vi "Periodic Tasks.vi"(8 "error in":errorcluster) -> ()   [LabVIEW 2017]
doc: "This VI runs in parallel to other tasks. It can contain as many user-defined periodic loops as you need. These can carry out PID or other sorts of timed response."
uses:
  <vilib>/Rock Robotics/WPI/Utilities/WPI_GetSetVariantRefNum.vi
  Robot Global Data.vi
  <vilib>/addons/control/pid/pid.llb/PID (DBL).vi
  <vilib>/Rock Robotics/WPI/RobotDrive/WPI_RobotDriveMecanumDrive_Cartesian.vi
  globals.vi
  <vilib>/addons/control/pid/NI_PID_pid.lvlib
  <vilib>/Rock Robotics/WPI/ThirdParty/Sensors/navX/_TypeDefs/FRIC_navX_DeviceNumbersTypeDef.ctl
panel:
  out "Shoulder Low Home":bool
  out "Wrist Low Home":bool
  out "Wrist High Home":bool
  out "X and Y  axis":cluster{"Distance":dbl, "Distance":dbl}(graph)={"Distance"=0.0, "Distance"=-36.75}
  out "Proxy":dbl(graph)=0.412597614
  in  "PID gains":T1={"proportional gain (Kc)"=0.015, "integral time (Ti, min)"=0.00357142, "derivative time (Td, min)"=0.00089286} {"derivative time (Td, min)" step=1e-05 format="%.9f"; "integral time (Ti, min)" step=1e-05 format="%.9f"; "proportional gain (Kc)" step=0.05 format="%.9f"}
  in  "Wrist Encoder Recording Data":cluster{dbl, u32}[](array[cluster])=[{0.0, 106}, {0.0, 200}, {0.0, 304}, {0.0, 400}, {16.75, 500}, {68.5, 600}, {96.0, 700}, {106.5, 800}, {112.5, 901}, {119.25, 1001}, {122.75, 1100}, {123.25, 1200}, {136.25, 1300}, {146.0, 1400}, {162.75, 1503}, {181.0, 1601}, {204.5, 1704}, {237.75, 1804}, {283.75, 1904}, {329.75, 2004}, {337.25, 2106}, {328.75, 2205}, {322.25, 2306}, {344.0, 2407}, {382.75, 2507}, {432.25, 2607}, {486.75, 2707}, {538.5, 2807}, {587.5, 2907}, {630.0, 3007}, {668.25, 3107}, {702.0, 3207}, {735.25, 3307}, {755.0, 3407}, {765.5, 3508}, {770.25, 3608}, {781.25, 3708}, {805.5, 3808}, {842.0, 3909}, {884.75, 4009}, {920.75, 4109}, {945.25, 4209}, {954.5, 4311}, {954.5, 4411}, {955.75, 4509}, {956.25, 4611}, {956.25, 4709}, {956.25, 4809}, {956.25, 4910}, {956.25, 5009}, {956.25, 5109}, {956.25, 5210}, {956.5, 5315}, {956.5, 5416}, {956.5, 5516}, {956.5, 5618}, {956.5, 5717}, {956.5, 5816}, {956.5, 5918}, {956.5, 6018}, {956.5, 6119}, {956.5, 6218}, {956.5, 6318}, {956.5, 6417}, {956.5, 6517}, {956.5, 6619}, {956.5, 6715}, {956.5, 6816}, {956.5, 6919}, {956.5, 7020}, {956.5, 7118}, {956.5, 7222}, {956.5, 7318}, {956.5, 7418}, {956.5, 7519}, {956.5, 7619}, {956.5, 7719}, {956.5, 7819}, {956.5, 7919}, {956.5, 8020}, {956.5, 8120}, {956.5, 8221}, {956.5, 8320}, {956.5, 8420}, {956.5, 8520}, {956.5, 8620}, {956.5, 8720}, {956.5, 8822}, {956.5, 8921}, {956.5, 9023}, {956.5, 9124}, {956.5, 9223}, {956.5, 9321}, {956.5, 9425}, {956.5, 9523}, {956.5, 9626}, {956.5, 9723}, {956.5, 9824}, {956.5, 9924}, {956.5, 10024}, {956.5, 10124}, {956.5, 10224}, {956.5, 10324}, {956.5, 10424}, {956.5, 10526}, {956.5, 10625}, {956.5, 10727}, {956.5, 10826}, {956.5, 10928}, {956.5, 11027}, {956.5, 11128}, {956.5, 11227}, {956.5, 11327}, {956.5, 11427}, {956.5, 11527}, {956.5, 11628}, {956.5, 11729}, {956.5, 11828}, {956.5, 11928}, {956.5, 12028}, {956.5, 12128}, {956.5, 12228}, {956.5, 12328}, {956.5, 12428}, {956.5, 12528}, {956.5, 12628}, {956.5, 12728}, {956.5, 12828}, {956.5, 12928}, {956.5, 13028}, {956.5, 13129}, {956.5, 13228}, {956.5, 13328}, {956.5, 13428}, {956.5, 13528}, {956.5, 13628}, {956.5, 13728}, {956.5, 13828}, {956.5, 13928}, {956.5, 14028}, {956.5, 14128}, {956.5, 14228}, {956.5, 14328}, {956.5, 14428}, {956.5, 14528}, {956.5, 14628}, {956.5, 14728}, {956.5, 14829}, {956.5, 14929}, {956.5, 15031}, {956.5, 15130}, {956.5, 15230}, {956.5, 15330}, {956.5, 15437}, {956.5, 15530}, {956.5, 15630}, {956.5, 15730}, {956.5, 15830}, {956.5, 15930}, {956.75, 16039}, {956.75, 16132}, {956.75, 16235}, {956.75, 16333}, {956.75, 16436}, {956.75, 16535}, {956.75, 16635}, {956.75, 16737}, {956.75, 16834}, {956.75, 16937}, {956.75, 17038}, {956.75, 17136}, {956.75, 17235}, {956.75, 17335}, {956.75, 17438}, {956.75, 17539}, {956.75, 17638}, {956.75, 17740}, {956.75, 17839}, {956.75, 17941}, {956.75, 18038}, {956.75, 18140}, {956.75, 18239}, {956.75, 18341}, {956.75, 18438}, {957.0, 18538}, {957.0, 18639}, {957.0, 18741}, {955.5, 18839}, {952.25, 18943}, {946.5, 19039}, {931.25, 19144}, {903.75, 19240}, {876.75, 19342}, {866.75, 19440}, {844.5, 19545}, {812.0, 19642}, {775.0, 19740}, {734.0, 19843}, {694.5, 19943}, {654.0, 20041}, {608.5, 20141}, {557.75, 20243}, {505.75, 20344}, {454.0, 20445}, {401.25, 20547}, {349.75, 20646}, {297.0, 20746}, {243.5, 20846}, {187.0, 20948}, {131.5, 21046}, {79.0, 21149}, {34.75, 21246}, {-9.25, 21349}, {-50.0, 21447}, {-92.0, 21547}, {-133.75, 21647}, {-175.75, 21747}, {-217.25, 21847}, {-259.75, 21947}, {-296.25, 22047}, {-317.25, 22148}, {-328.75, 22248}, {-354.75, 22348}, {-404.0, 22449}, {-466.75, 22549}, {-535.5, 22649}, {-606.25, 22749}, {-666.0, 22849}, {-716.75, 22949}, {-768.25, 23052}, {-816.75, 23149}, {-854.25, 23250}, {-886.5, 23349}, {-924.75, 23453}, {-962.75, 23549}, {-996.25, 23650}, {-1021.25, 23749}, {-1043.75, 23850}, {-1066.25, 23949}, {-1089.25, 24050}, {-1114.0, 24153}, {-1137.25, 24251}, {-1163.25, 24352}, {-1190.25, 24455}, {-1216.5, 24556}, {-1239.5, 24657}, {-1261.0, 24758}, {-1273.25, 24856}, {-1274.0, 24957}, {-1274.0, 25057}, {-1274.0, 25157}, {-1278.5, 25258}, {-1295.5, 25361}, {-1317.25, 25460}, {-1344.25, 25560}, {-1372.0, 25660}, {-1389.75, 25757}, {-1402.0, 25859}, {-1411.0, 25960}, {-1419.75, 26060}, {-1427.0, 26163}, {-1430.5, 26260}]
  in  "Shoulder Encoder Recording Data":cluster{dbl, u32}[](array[cluster])=[{0.0, 107}, {0.0, 200}, {0.0, 304}, {0.0, 400}, {0.0, 500}, {0.0, 600}, {0.0, 700}, {0.0, 800}, {0.0, 901}, {0.0, 1001}, {0.0, 1100}, {0.0, 1200}, {0.0, 1300}, {0.0, 1400}, {0.0, 1502}, {0.0, 1601}, {0.0, 1704}, {0.0, 1805}, {0.0, 1904}, {0.0, 2004}, {0.0, 2106}, {0.0, 2205}, {0.0, 2306}, {0.0, 2407}, {0.0, 2507}, {0.0, 2607}, {0.0, 2707}, {0.0, 2807}, {0.0, 2907}, {0.0, 3007}, {0.0, 3107}, {0.0, 3207}, {0.0, 3307}, {0.0, 3408}, {0.0, 3508}, {0.0, 3608}, {0.0, 3708}, {0.0, 3808}, {0.0, 3909}, {0.0, 4009}, {0.0, 4109}, {0.0, 4209}, {0.0, 4309}, {0.0, 4412}, {0.0, 4509}, {0.0, 4618}, {0.0, 4709}, {0.0, 4809}, {0.0, 4911}, {0.0, 5009}, {0.0, 5109}, {0.0, 5210}, {0.0, 5314}, {-32.5, 5417}, {-235.75, 5517}, {-410.5, 5618}, {-521.25, 5717}, {-594.5, 5816}, {-669.0, 5919}, {-733.25, 6018}, {-810.25, 6119}, {-896.75, 6218}, {-986.5, 6318}, {-1072.0, 6417}, {-1157.0, 6517}, {-1247.75, 6619}, {-1339.75, 6716}, {-1440.75, 6816}, {-1550.25, 6919}, {-1659.5, 7020}, {-1763.0, 7118}, {-1872.75, 7223}, {-1969.75, 7318}, {-2070.0, 7418}, {-2177.25, 7519}, {-2285.25, 7619}, {-2392.5, 7719}, {-2500.5, 7819}, {-2609.0, 7919}, {-2722.5, 8020}, {-2837.5, 8120}, {-2960.25, 8221}, {-3080.75, 8320}, {-3214.75, 8420}, {-3339.75, 8520}, {-3472.5, 8620}, {-3603.25, 8720}, {-3742.75, 8822}, {-3871.0, 8921}, {-4011.0, 9023}, {-4146.25, 9124}, {-4282.0, 9224}, {-4417.0, 9322}, {-4559.5, 9425}, {-4695.75, 9523}, {-4839.5, 9626}, {-4986.0, 9723}, {-5140.25, 9824}, {-5301.25, 9924}, {-5459.5, 10024}, {-5617.75, 10124}, {-5775.5, 10224}, {-5924.25, 10324}, {-6078.75, 10424}, {-6241.5, 10527}, {-6406.75, 10626}, {-6582.0, 10727}, {-6765.25, 10826}, {-6960.5, 10928}, {-7157.25, 11027}, {-7359.75, 11128}, {-7549.25, 11227}, {-7743.75, 11327}, {-7936.75, 11427}, {-8133.0, 11527}, {-8339.0, 11628}, {-8545.25, 11729}, {-8752.25, 11828}, {-8964.0, 11928}, {-9184.75, 12028}, {-9406.0, 12128}, {-9634.25, 12228}, {-9863.25, 12328}, {-10093.25, 12428}, {-10323.75, 12528}, {-10567.5, 12628}, {-10814.0, 12728}, {-11069.0, 12829}, {-11321.75, 12928}, {-11576.75, 13028}, {-11843.0, 13129}, {-12103.5, 13228}, {-12375.25, 13328}, {-12657.25, 13428}, {-12940.25, 13528}, {-13223.0, 13628}, {-13516.0, 13728}, {-13813.5, 13828}, {-14115.0, 13928}, {-14420.5, 14028}, {-14726.75, 14128}, {-15036.0, 14228}, {-15351.25, 14328}, {-15664.0, 14428}, {-16003.0, 14528}, {-16336.75, 14628}, {-16681.75, 14728}, {-17028.25, 14829}, {-17378.75, 14929}, {-17738.75, 15030}, {-18102.0, 15130}, {-18471.25, 15230}, {-18833.5, 15330}, {-19231.5, 15436}, {-19593.0, 15530}, {-19983.0, 15631}, {-20375.75, 15730}, {-20776.0, 15830}, {-21183.25, 15930}, {-21620.5, 16036}, {-22020.5, 16132}, {-22450.75, 16234}, {-22877.75, 16333}, {-23288.5, 16437}, {-23583.0, 16535}, {-23844.5, 16635}, {-24068.0, 16737}, {-24254.75, 16835}, {-24444.5, 16937}, {-24614.25, 17038}, {-24785.75, 17137}, {-25022.25, 17235}, {-25292.25, 17335}, {-25618.25, 17438}, {-25956.75, 17537}, {-26300.75, 17638}, {-26631.75, 17738}, {-26913.25, 17839}, {-27134.25, 17941}, {-27312.75, 18038}, {-27499.75, 18140}, {-27676.25, 18239}, {-27797.0, 18341}, {-27874.5, 18438}, {-27944.5, 18538}, {-28058.75, 18639}, {-28186.5, 18741}, {-28280.75, 18839}, {-28331.0, 18943}, {-28353.25, 19039}, {-28372.25, 19144}, {-28372.25, 19240}, {-28372.25, 19341}, {-28372.5, 19440}, {-28372.5, 19544}, {-28372.5, 19642}, {-28373.25, 19740}, {-28378.5, 19843}, {-28400.75, 19943}, {-28506.25, 20041}, {-28714.0, 20142}, {-28955.5, 20243}, {-29241.0, 20345}, {-29553.5, 20445}, {-29899.75, 20547}, {-30260.5, 20645}, {-30661.25, 20746}, {-31071.5, 20846}, {-31526.25, 20948}, {-32031.0, 21046}, {-32581.5, 21149}, {-33082.0, 21246}, {-33630.0, 21349}, {-34199.75, 21447}, {-34815.0, 21548}, {-35462.25, 21647}, {-36093.25, 21747}, {-36734.75, 21847}, {-37431.0, 21948}, {-38130.25, 22047}, {-38593.5, 22148}, {-38803.75, 22248}, {-39030.75, 22348}, {-39233.5, 22449}, {-39362.0, 22549}, {-39440.75, 22649}, {-39492.75, 22749}, {-39529.0, 22849}, {-39548.5, 22949}, {-39577.5, 23052}, {-39693.75, 23150}, {-39876.0, 23250}, {-40038.25, 23349}, {-40102.5, 23455}, {-40103.0, 23549}, {-40103.0, 23650}, {-40103.0, 23749}, {-40103.0, 23850}, {-40103.0, 23949}, {-40103.0, 24049}, {-40103.0, 24157}, {-40103.0, 24252}, {-40103.0, 24351}, {-40103.0, 24455}, {-40103.0, 24556}, {-40103.0, 24656}, {-40103.0, 24758}, {-40103.0, 24856}, {-40103.0, 24957}, {-40103.0, 25057}, {-40103.0, 25157}, {-40103.0, 25259}, {-40103.0, 25362}, {-40103.0, 25460}, {-40103.0, 25560}, {-40103.0, 25660}, {-40103.0, 25757}, {-40103.0, 25859}, {-40103.0, 25960}, {-40103.0, 26060}, {-40103.0, 26161}, {-40103.0, 26260}]
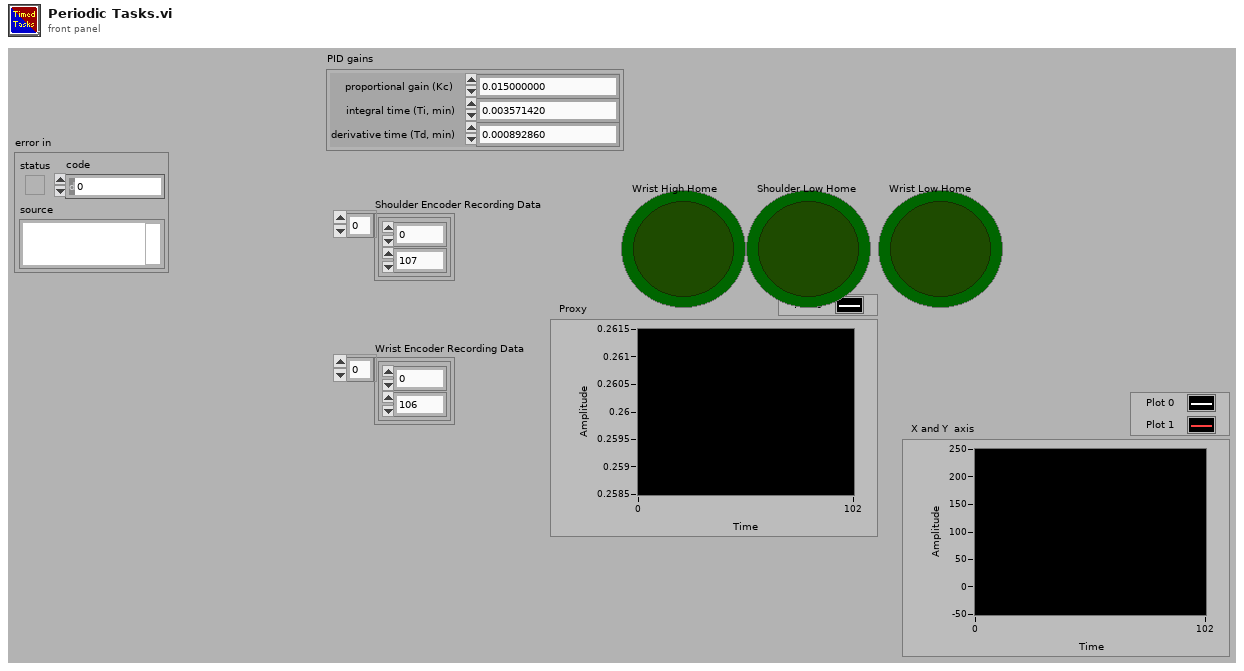
[diagram p1: front panel]
types:
  T1 = cluster{"proportional gain (Kc)":dbl, "integral time (Ti, min)":dbl, "derivative time (Td, min)":dbl}
  T2 = cluster{"Yaw":dbl, "Roll":dbl, "Pitch":dbl, "Heading":dbl, "Fused Heading":dbl}
  T3 = typedef "WPI_JoystickDevRef.ctl" = cluster{"Device":T4}
  T4 = typedef "WPI_JoystickDeviceEnum.ctl" = enum16{"USB 0", "USB 1", "USB 2", "USB 3", "USB 4", "USB 5"}
  T5 = typedef "WPI_EncoderDevRef.ctl" = cluster{"DevStatus":errorcluster, "EncoderIndex":T6, "CounterIndex":T7, "DistancePerCount":dbl, "Decoding Type":T8}
  T6 = typedef "FPGA_EncoderIdx.ctl" = enum8{"Enc 0", "Enc 1", "Enc 2", "Enc 3", "Enc 4", "Enc 5", "Enc 6", "Enc 7", "Invalid"}
  T7 = typedef "FPGA_CounterCtrSystemIndex.ctl" = enum8{"Ctr 0", "Ctr 1", "Ctr 2", "Ctr 3", "Ctr 4", "Ctr 5", "Ctr 6", "Ctr 7", "Invalid"}
  T8 = typedef "WPI_EncoderType.ctl" = enum16{"1x", "2x", "4x"}
  T9 = cluster{"Motor Selection":string, "EncoderDevRef":T5}
  T10 = typedef "FRIC_navX_DeviceNumbersTypeDef.ctl" = enum16{"Dev0", "Dev1", "Dev2", "Dev3"}
  T11 = typedef "WPI_RobotDriveDevRef.ctl" = cluster{"DevStatus":errorcluster, "Motors[]":T12[], "Square Inputs":bool, "Max Output":dbl}
  T12 = typedef "WPI_MotorControlDeviceRef.ctl" = cluster{"DeviceStatus":errorcluster, "Type":T13, "PWM":cluster{"PWM Channel":T14, "DeadBand":T15}, "CAN":cluster{"Device Number":u8, "SetOutput VI Ref":variant, "GetOutput VI Ref":variant, "Enable VI Ref":variant, "Disable VI Ref":variant, "Data":variant}, "Invert":bool, "DIO PWM":cluster{"PWM \"Enable\" Channel":T14, "DIOChannel":T16, "PWM Rate":dbl}}
  T13 = typedef "WPI_MotorControlType.ctl" = enum16{"PWM", "CAN", "DIO PWM"}
  T14 = typedef "FPGA_DIOPWMChannel.ctl" = enum8{"PWM 0", "PWM 1", "PWM 2", "PWM 3", "PWM 4", "PWM 5", "PWM 6", "PWM 7", "PWM 8", "PWM 9", "PWM MXP 0", "PWM MXP 1", "PWM MXP 2", "PWM MXP 3", "PWM MXP 4", "PWM MXP 5", "PWM MXP 6", "PWM MXP 7", "PWM MXP 8", "PWM MXP 9", "Invalid"}
  T15 = typedef "WPI_PWMDeadband.ctl" = cluster{"Name":string, "maxPositivePwm":i32, "minPositivePwm":i32, "centerPwm":i32, "maxNegativePwm":i32, "minNegativePwm":i32, "angularRange":u16}
  T16 = typedef "FPGA_DIOChannel.ctl" = enum8{"DIO 0", "DIO 1", "DIO 2", "DIO 3", "DIO 4", "DIO 5", "DIO 6", "DIO 7", "DIO 8", "DIO 9", "DIO MXP 0", "DIO MXP 1", "DIO MXP 2", "DIO MXP 3", "DIO MXP 4", "DIO MXP 5", "DIO MXP 6", "DIO MXP 7", "DIO MXP 8", "DIO MXP 9", "DIO MXP 10", "DIO MXP 11", "DIO MXP 12", "DIO MXP 13", "DIO MXP 14", "DIO MXP 15", "SPI Port CS1", "SPI Port CS2", "SPI Port CS3", "SPI Port MISO", "SPI Port MOSI", "Invalid"}
  T17 = cluster{"JoystickDevRef":T3, "RobotDriveDevRef":T11}
  T18 = typedef "WPI_DriverStationRobotMode2.ctl" = enum16{"Autonomous Disabled", "Autonomous Enabled", "Teleop Disabled", "Teleop Enabled", "Disconnected", "Finish", "Test Disabled", "Test Enabled", "Emergency Stopped"}
  T19 = typedef "WPI_AnalogChannelDevRef.ctl" = cluster{"DevStatus":errorcluster, "Analog Channel":T20}
  T20 = typedef "FPGA_AIChannel.ctl" = enum8{"AI 0", "AI 1", "AI 2", "AI 3", "AI MXP 0", "AI MXP 1", "AI MXP 2", "AI MXP 3", "Invalid"}
  T21 = typedef "WPI_DigitalInputDevRef.ctl" = cluster{"DevStatus":errorcluster, "DIO Channel":T16}
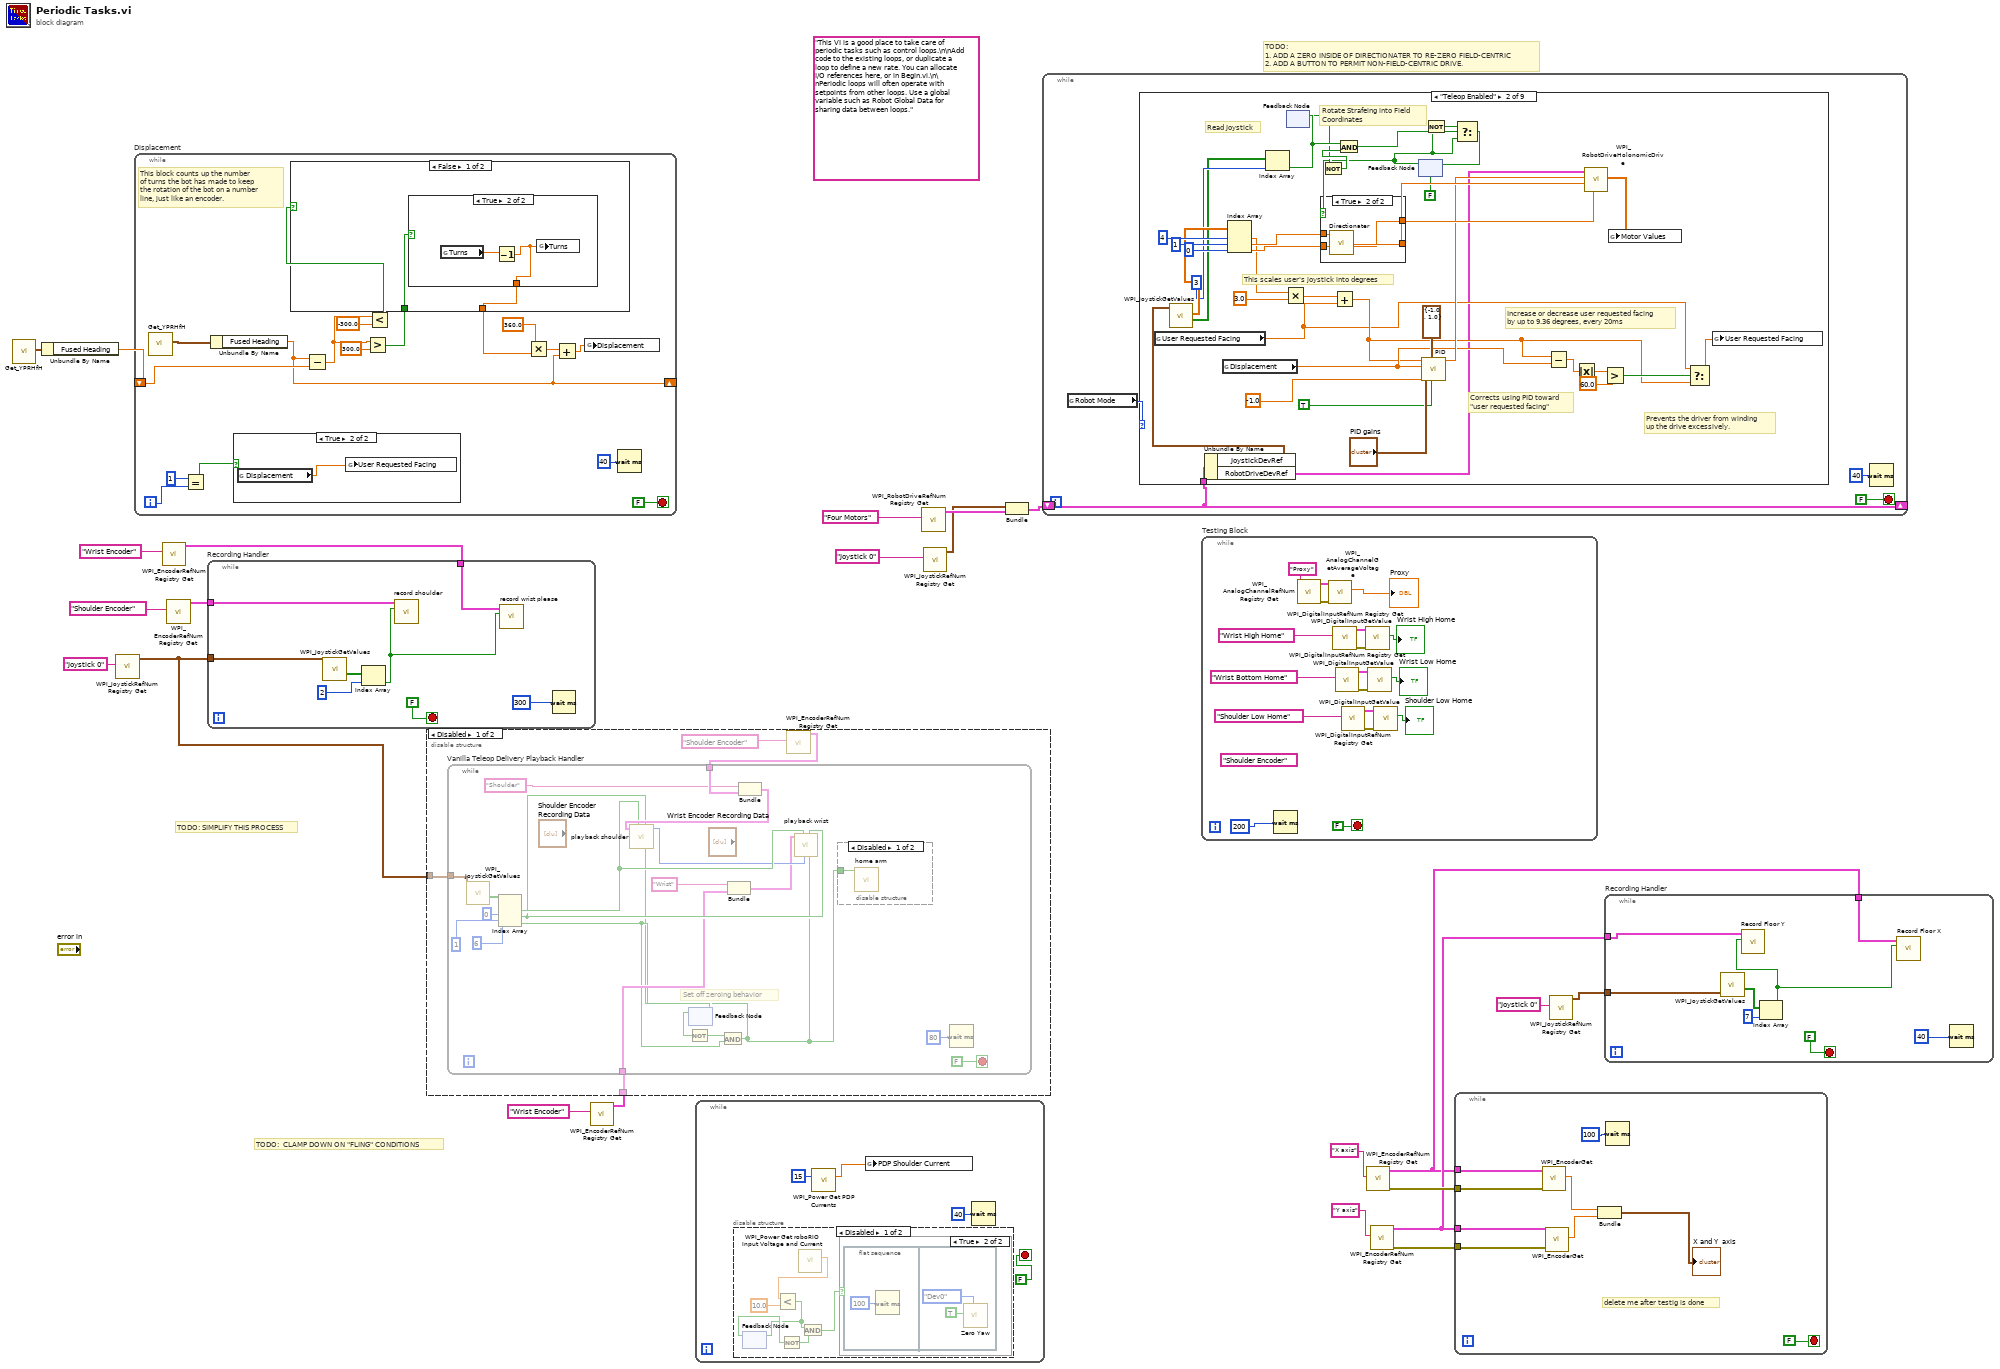
[diagram p0: block diagram]
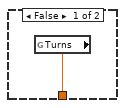
[diagram p3: hidden frame]
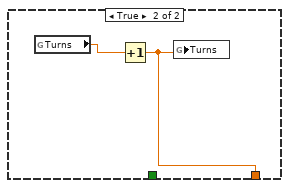
[diagram p4: hidden frame]
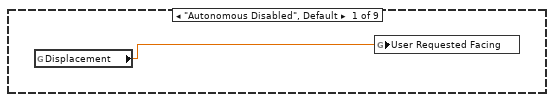
[diagram p9: hidden frame]
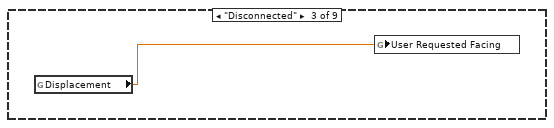
[diagram p11: hidden frame]
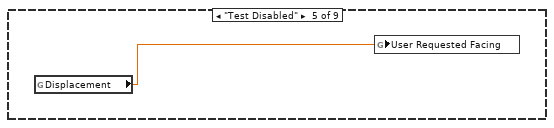
[diagram p13: hidden frame]
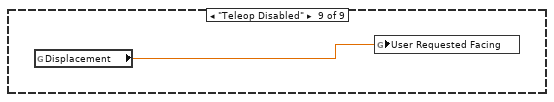
[diagram p17: hidden frame]
diagram:
  (unwired) "This VI is a good place to take care of periodic tasks such as control loops.\n\nAdd code to the existing loops, or duplicate a loop to define a new rate. You can allocate I/O references here, or in Begin.vi.\n\nPeriodic loops will often operate with setpoints from other loops. Use a global variable such as Robot Global Data for sharing data between loops."
  # "TODO:\n1. ADD A ZERO INSIDE OF DIRECTIONATER TO RE-ZERO FIELD-CENTRIC\n2. ADD A BUTTON TO PERMIT NON-FIELD-CENTRIC DRIVE."
  # "TODO:  CLAMP DOWN ON \"FLING\" CONDITIONS"
  # "TODO: SIMPLIFY THIS PROCESS"
  n1 = call <vilib>:"Get_YPRHfH.vi"() -> ("YRPHfH"=w1:T2)  [unwired: 11 in]
  n2 = Unbundle By Name(w1) -> ("Fused Heading"=w2:dbl)
  n3 = call <vilib>:"WPI_JoystickRefNum Registry Get.vi"("refnum name"="Joystick 0") -> ("JoystickDevRef"=w13:T3)  [unwired: 1 in, 9 out]
  n4 = while "Displacement" {
    shift-right: [w34] -> _
    shift-left: w2 -> [w38]
    i -> [w26]
    stop <- FALSE stop-if-true
    # "This block counts up the number\nof turns the bot has made to keep\nthe rotation of the bot on a number\nline, just like an encoder."
    n5 = call <vilib>:"Get_YPRHfH.vi"() -> ("YRPHfH"=w40:T2)  [unwired: 11 in]
    n6 = Equal?(x=1, y=w26) -> (x = y?=w24:bool)
    n7 = Unbundle By Name(w40) -> ("Fused Heading"=w34:dbl)
    n8 = case shown="True" w24 {
      frame False {
      }
      frame True {
        n9 = global read "Robot Global Data.vi" "Displacement"() -> (w41:dbl)
        n10 = global write "Robot Global Data.vi" "User Requested Facing"(w41) -> ()
      }
    }
    n11 = Subtract(x=w34, y=w38) -> (x-y=w30:dbl)
    n12 = Greater?(x=w30, y=300.0 ("x")) -> (0:w28:bool)
    n13 = Less?(x=w30, y=-300.0) -> (x < y?=w37:bool)
    n14 = case shown="False" w37 {
      tunnel: w28 -> [w43 _]
      tunnel: [w42 w47] -> w27
      frame False {
        n15 = case shown="True" w43 {
          tunnel: [w44 w45] -> w42
          frame False {
            n16 = global read "Robot Global Data.vi" "Turns"() -> (w44:dbl)
          }
          frame True {
            n17 = global read "Robot Global Data.vi" "Turns"() -> (w46:dbl)
            n18 = Decrement(x=w46) -> (x-1=w45:dbl)
            n19 = global write "Robot Global Data.vi" "Turns"(w45) -> ()
          }
        }
      }
      frame True {
        n20 = global read "Robot Global Data.vi" "Turns"() -> (w48:dbl)
        n21 = Increment(x=w48) -> (x+1=w47:dbl)
        n22 = global write "Robot Global Data.vi" "Turns"(w47) -> ()
      }
    }
    n23 = Multiply(x=360.0, y=w27) -> (x*y=w35:dbl)
    n24 = Add(x=w35, y=w34) -> (x+y=w33:dbl)
    n25 = global write "Robot Global Data.vi" "Displacement"(w33) -> ()
    n26 = Wait (ms)(milliseconds to wait=u32 40) -> ()  [unwired: 1 out]
  }
  n27 = call <vilib>:"WPI_EncoderRefNum Registry Get.vi"("refnum name"="Wrist Encoder") -> ("EncoderDevRef"=w19:T5)  [unwired: 9 in, 1 out]
  n28 = call <vilib>:"WPI_EncoderRefNum Registry Get.vi"("refnum name"="Shoulder Encoder") -> ("EncoderDevRef"=w21:T5)  [unwired: 9 in, 1 out]
  n29 = while "Recording Handler" {
    tunnel: w21 -> [w53]
    tunnel: w19 -> [w52]
    tunnel: w13 -> [w51]
    stop <- FALSE stop-if-true
    n30 = call <vilib>:"WPI_JoystickGetValues.vi"("JoystickDevRef"=w51) -> ("Buttons"=w54:bool[])  [unwired: 6 in, 4 out]
    n31 = Index Array(array=w54, index=2) -> (element=w49:bool)
    n32 = call "record shoulder.vi"("Record"=w49, "EncoderDevRef"=w53) -> ()  [unwired: 7 in, 2 out]
    n33 = call "record wrist please.vi"("Record"=w49, "EncoderDevRef"=w52) -> ()  [unwired: 7 in, 2 out]
    n34 = Wait (ms)(milliseconds to wait=u32 300) -> ()  [unwired: 1 out]
  }
  n35 = call <vilib>:"WPI_EncoderRefNum Registry Get.vi"("refnum name"="Wrist Encoder") -> ("EncoderDevRef"=w11:T5)  [unwired: 9 in, 1 out]
  n36 = disable-structure shown="Disabled" {
    disable-tunnel: w13 -> [w60 _]
    disable-tunnel: w11 -> [w57 _]
    frame Disabled {
      n37 = call <vilib>:"WPI_EncoderRefNum Registry Get.vi"("refnum name"="Shoulder Encoder") -> ("EncoderDevRef"=w58:T5)  [unwired: 9 in, 1 out]
      n38 = while "Vanilla Teleop Delivery Playback Handler" {
        tunnel: w58 -> [w75]
        tunnel: w60 -> [w70]
        tunnel: w57 -> [w69]
        stop <- FALSE stop-if-true
        # "Set off zeroing behavior"
        n39 = call <vilib>:"WPI_JoystickGetValues.vi"("JoystickDevRef"=w70) -> ("Buttons"=w80:bool[])  [unwired: 6 in, 4 out]
        n40 = Index Array(array=w80, index #1=0 ("index"), index #2=1 ("index"), index #3=6 ("index")) -> (element #1=w72:bool, element #2=w71:bool, element #3=w67:bool)
        n41 = feedback-in #1(w67) -> ()
        n42 = feedback #1() -> (w65:bool)  [unwired: 1 in]
        n43 = Not(x=w65) -> (.not. x?=w66:bool)
        n44 = And(x=w66, y=w67) -> (x .and. y?=w64:bool)
        n45 = Bundle("Motor Selection"="Wrist", "EncoderDevRef"=w69) -> (w61:T9)  [unwired: 1 in]
        n46 = Bundle("Motor Selection"="Shoulder", "EncoderDevRef"=w75) -> (w76:T9)  [unwired: 1 in]
        n47 = call "playback shoulder.vi"("Home"=w64, "Rewind"=w71, "Playback"=w72, "Hardware In"=w76) -> ("Encoder Frame"=w62:i32)  [unwired: 6 in, 1 out]
        n48 = call "playback wrist.vi"("Home"=w64, "Rewind"=w71, "Encoder Frame"=w62, "Playback"=w72, "Hardware In"=w61) -> ()  [unwired: 6 in, 1 out]
        n49 = disable-structure shown="Disabled" {
          disable-tunnel: w64 -> [w81 _]
          frame Disabled {
            n50 = call "home arm.vi"("Home"=w81) -> ()  [unwired: 11 in]
          }
          frame Enabled {
          }
        }
        n51 = Wait (ms)(milliseconds to wait=u32 80) -> ()  [unwired: 1 out]
      }
    }
    frame Enabled {
    }
  }
  n52 = while {
    stop <- FALSE stop-if-true
    n53 = disable-structure shown="Disabled" {
      frame Disabled {
        n54 = feedback #2() -> (w88:bool)  [unwired: 1 in]
        n55 = Not(x=w88) -> (.not. x?=w89:bool)
        n56 = call <vilib>:"WPI_Power Get roboRIO Input Voltage and Current.vi"() -> ("roboRIO input voltage (V)"=w91:dbl)  [unwired: 13 in, 2 out]
        n57 = Less?(x=w91, y=10.0) -> (x < y?=w87:bool)
        n58 = feedback-in #2(w87) -> ()
        n59 = And(x=w87, y=w89) -> (x .and. y?=w86:bool)
        n60 = case shown="True" w86 {
          frame False {
          }
          frame True {
            n61 = flat-sequence {
              frame #0 {
                n62 = Wait (ms)(milliseconds to wait=u32 100) -> ()  [unwired: 1 out]
              }
              frame #1 {
                n63 = call <vilib>:"Zero Yaw.vi"("Device Number"=FRIC_navX_DeviceNumbersTypeDef."Dev0", "Zero"=TRUE) -> ()  [unwired: 10 in]
              }
            }
          }
        }
      }
      frame Enabled {
      }
    }
    n64 = call <vilib>:"WPI_Power Get PDP Currents.vi"("PDP Channel"=15) -> ("current (A)"=w83:dbl)  [unwired: 12 in, 2 out]
    n65 = global write "globals.vi" "PDP Shoulder Current"(w83) -> ()
    n66 = Wait (ms)(milliseconds to wait=u32 40) -> ()  [unwired: 1 out]
  }
  n67 = call <vilib>:"WPI_RobotDriveRefNum Registry Get.vi"("refnum name"="Four Motors") -> ("RobotDriveDevRef"=w16:T11)  [unwired: 9 in, 1 out]
  n68 = call <vilib>:"WPI_JoystickRefNum Registry Get.vi"("refnum name"="Joystick 0") -> ("JoystickDevRef"=w15:T3)  [unwired: 9 in, 1 out]
  n69 = Bundle("JoystickDevRef"=w15, "RobotDriveDevRef"=w16) -> (w14:T17)  [unwired: 1 in]
  n70 = while {
    shift-right: [w95] -> _
    shift-left: w14 -> [w95]
    stop <- FALSE stop-if-true
    n71 = global read "Robot Global Data.vi" "Robot Mode"() -> (w96:T18)
    n72 = case shown="\"Teleop Enabled\"" w96 {
      tunnel: w95 -> [_ w137 _ _ _ _ _ _ _]
      frame "Autonomous Disabled", Default {
        n73 = global read "Robot Global Data.vi" "Displacement"() -> (w99:dbl)
        n74 = global write "Robot Global Data.vi" "User Requested Facing"(w99) -> ()
      }
      frame "Teleop Enabled" {
        # "Prevents the driver from winding\nup the drive excessively."
        # "This scales user's joystick into degrees"
        # "Increase or decrease user requested facing\nby up to 9.36 degrees, every 20ms"
        # "Corrects using PID toward\n\"user requested facing\""
        # "Rotate Strafeing into Field\nCoordinates"
        # "Read Joystick"
        n75 = global read "Robot Global Data.vi" "User Requested Facing"() -> (w112:dbl)
        n76 = Unbundle By Name(w137) -> ("JoystickDevRef"=w131:T3, "RobotDriveDevRef"=w100:T11)
        n77 = call <vilib>:"WPI_JoystickGetValues.vi"("JoystickDevRef"=w131) -> ("Buttons"=w109:bool[], "Axes"=w130:dbl[])  [unwired: 6 in, 3 out]
        n78 = global read "Robot Global Data.vi" "Displacement"() -> (w117:dbl)
        n79 = Index Array(array=w130, index #1=4 ("index"), index #2=1 ("index"), index #3=0 ("index")) -> (element #1=w122:dbl, element #2=w133:dbl, element #3=w132:dbl)
        n80 = Index Array(array=w109, index=3) -> (element=w107:bool)
        n81 = Multiply(x=w122, y=3.0) -> (x*y=w120:dbl)
        n82 = feedback-in #3(w107) -> ()
        n83 = feedback #3() -> (w106:bool)  [unwired: 1 in]
        n84 = Not(x=w106) -> (.not. x?=w108:bool)
        n85 = Add(x=w120, y=w112) -> (x+y=w113:dbl)
        n86 = And(x=w107, y=w108) -> (x .and. y?=w104:bool)
        n87 = feedback #4(FALSE) -> (w101:bool)
        n88 = case shown="True" w101 {
          tunnel: w133 -> [w138 w143]
          tunnel: w132 -> [w139 w142]
          tunnel: [w138 w141] -> w125
          tunnel: [w139 w140] -> w124
          frame False {
          }
          frame True {
            n89 = call "Directionater.vi"("Y In"=w142, "X In"=w143) -> ("Y"=w140:dbl, "Rotation"=w141:dbl)  [unwired: 8 in]
          }
        }
        n90 = call-poly <vilib>:"PID.vi"("reinitialize? (F)"=TRUE, "output range"=cluster{"output low":dbl, "output high":dbl} {"output low"=-1.0, "output high"=1.0}, "dt (s)"=-1.0, "PID gains"="PID gains", "process variable"=w117, "setpoint"=w113) -> ("output"=w123:dbl)  [unwired: 4 in, 1 out]
        n91 = Not(x=w101) -> (.not. x?=w103:bool)
        n92 = Select(t=w103, s=w104, f=w101) -> (s? t:f=w102:bool)
        n93 = feedback-in #4(w102) -> ()
        n94 = Subtract(x=w113, y=w117) -> (x-y=w119:dbl)
        n95 = Absolute Value(x=w119) -> (abs(x)=w118:dbl)
        n96 = call-poly <vilib>:"WPI_RobotDriveHolonomicDrive.vi"("Rotation"=w124, "Y"=w125, "X"=w123, "RobotDriveDevRef"=w100) -> ("Motor Values"=w111:dbl[])  [unwired: 5 in, 2 out]
        n97 = Greater?(x=w118, y=60.0) -> (0:w115:bool)
        n98 = global write "Robot Global Data.vi" "Motor Values"(w111) -> ()
        n99 = Select(t=w112, s=w115, f=w113) -> (s? t:f=w114:dbl)
        n100 = global write "Robot Global Data.vi" "User Requested Facing"(w114) -> ()
      }
      frame "Disconnected" {
        n101 = global read "Robot Global Data.vi" "Displacement"() -> (w144:dbl)
        n102 = global write "Robot Global Data.vi" "User Requested Facing"(w144) -> ()
      }
      frame "Finish" {
      }
      frame "Test Disabled" {
        n103 = global read "Robot Global Data.vi" "Displacement"() -> (w145:dbl)
        n104 = global write "Robot Global Data.vi" "User Requested Facing"(w145) -> ()
      }
      frame "Test Enabled" {
      }
      frame "Emergency Stopped" {
      }
      frame "Autonomous Enabled" {
      }
      frame "Teleop Disabled" {
        n105 = global read "Robot Global Data.vi" "Displacement"() -> (w146:dbl)
        n106 = global write "Robot Global Data.vi" "User Requested Facing"(w146) -> ()
      }
    }
    n107 = Wait (ms)(milliseconds to wait=u32 40) -> ()  [unwired: 1 out]
  }
  n108 = while "Testing Block" {
    stop <- FALSE stop-if-true
    (unwired) "Shoulder Encoder" ("refnum name")
    n109 = Wait (ms)(milliseconds to wait=u32 200) -> ()  [unwired: 1 out]
    n110 = call <vilib>:"WPI_AnalogChannelRefNum Registry Get.vi"("refnum name"="Proxy") -> ("error out"=w160:errorcluster, "AIDeviceRef"=w161:T19)  [unwired: 9 in]
    n111 = call <vilib>:"WPI_AnalogChannelGetAverageVoltage.vi"("error in (no error)"=w160, "AIDeviceRef"=w161) -> ("Voltage"=→"Proxy":dbl)  [unwired: 7 in, 2 out]
    n112 = call <vilib>:"WPI_DigitalInputRefNum Registry Get.vi"("refnum name"="Wrist High Home") -> ("error out"=w157:errorcluster, "DigitalInputDevRef"=w156:T21)  [unwired: 9 in]
    n113 = call <vilib>:"WPI_DigitalInputRefNum Registry Get.vi"("refnum name"="Wrist Bottom Home") -> ("error out"=w153:errorcluster, "DigitalInputDevRef"=w152:T21)  [unwired: 9 in]
    n114 = call <vilib>:"WPI_DigitalInputRefNum Registry Get.vi"("refnum name"="Shoulder Low Home") -> ("error out"=w149:errorcluster, "DigitalInputDevRef"=w148:T21)  [unwired: 9 in]
    n115 = call <vilib>:"WPI_DigitalInputGetValue.vi"("error in (no error)"=w157, "DigitalInputDevRef"=w156) -> ("Value"=→"Wrist High Home":bool)  [unwired: 7 in, 2 out]
    n116 = call <vilib>:"WPI_DigitalInputGetValue.vi"("error in (no error)"=w153, "DigitalInputDevRef"=w152) -> ("Value"=→"Wrist Low Home":bool)  [unwired: 7 in, 2 out]
    n117 = call <vilib>:"WPI_DigitalInputGetValue.vi"("error in (no error)"=w149, "DigitalInputDevRef"=w148) -> ("Value"=→"Shoulder Low Home":bool)  [unwired: 7 in, 2 out]
  }
  n118 = call <vilib>:"WPI_EncoderRefNum Registry Get.vi"("refnum name"="X axis") -> ("error out"=w8:errorcluster, "EncoderDevRef"=w4:T5)  [unwired: 9 in]
  n119 = call <vilib>:"WPI_EncoderRefNum Registry Get.vi"("refnum name"="Y axis") -> ("error out"=w7:errorcluster, "EncoderDevRef"=w5:T5)  [unwired: 9 in]
  n120 = while {
    tunnel: w8 -> [w168]
    tunnel: w4 -> [w167]
    tunnel: w7 -> [w166]
    tunnel: w5 -> [w165]
    stop <- FALSE stop-if-true
    # "delete me after testig is done"
    n121 = call <vilib>:"WPI_EncoderGet.vi"("error in (no error)"=w168, "EncoderDevRef"=w167) -> ("Distance"=w172:dbl)  [unwired: 4 in, 5 out]
    n122 = call <vilib>:"WPI_EncoderGet.vi"("error in (no error)"=w166, "EncoderDevRef"=w165) -> ("Distance"=w173:dbl)  [unwired: 4 in, 5 out]
    n123 = Bundle("Distance"=w172, "Distance"=w173) -> (→"X and Y  axis":cluster{"Distance":dbl, "Distance":dbl})  [unwired: 1 in]
    n124 = Wait (ms)(milliseconds to wait=u32 100) -> ()  [unwired: 1 out]
  }
  n125 = call <vilib>:"WPI_JoystickRefNum Registry Get.vi"("refnum name"="Joystick 0") -> ("JoystickDevRef"=w3:T3)  [unwired: 1 in, 9 out]
  n126 = while "Recording Handler" {
    tunnel: w5 -> [w177]
    tunnel: w4 -> [w174]
    tunnel: w3 -> [w178]
    stop <- FALSE stop-if-true
    n127 = call <vilib>:"WPI_JoystickGetValues.vi"("JoystickDevRef"=w178) -> ("Buttons"=w179:bool[])  [unwired: 6 in, 4 out]
    n128 = Index Array(array=w179, index=7) -> (element=w175:bool)
    n129 = call "Record Floor Y.vi"("Record"=w175, "EncoderDevRef"=w177) -> ()  [unwired: 7 in, 2 out]
    n130 = call "Record Floor X.vi"("Record"=w175, "EncoderDevRef"=w174) -> ()  [unwired: 7 in, 2 out]
    n131 = Wait (ms)(milliseconds to wait=u32 40) -> ()  [unwired: 1 out]
  }
